vi "Write Response to TCP.vi"(8 "error in (no error)":errorcluster, 9 "TCP Connection":refnum<k5>, 11 "Response in":refnum<class "Response.lvclass">) -> (0 "error out":errorcluster, 3 "Response out":refnum<class "Response.lvclass">)   [LabVIEW 2023, in "HTTP Utils.lvlib" / "Response.lvclass"]
uses:
  Response.lvclass
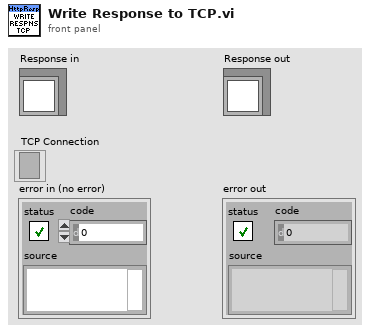
[diagram p1: front panel]
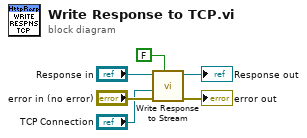
[diagram p0: block diagram]
diagram:
  n1 = call-dynamic "Write Response to Stream.vi"("Close? (T)"=FALSE, "error in (no error)"="error in (no error)", "Stream in"="TCP Connection", "Response in"="Response in") -> ("error out"=→"error out":errorcluster, "Response out"=→"Response out":refnum<class "Response.lvclass">)  [unwired: 6 in]
